vi "Exit.vi"(8 "error in (no error)":errorcluster, 11 "Door Controller in":refnum<class "Door Controller.lvclass">) -> (0 "error out":errorcluster, 3 "Door Controller out":refnum<class "Door Controller.lvclass">)   [LabVIEW 2020, in "Door Controller.lvlib" / "Door Controller.lvclass"]
uses:
  Door Controller.lvclass
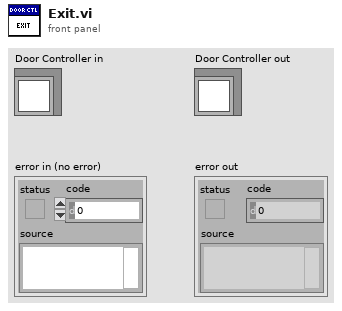
[diagram p1: front panel]
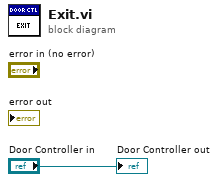
[diagram p0: block diagram]
diagram:
  "Door Controller out" <- "Door Controller in"
